vi "Main Page.vi"(8 "error in (no error)":errorcluster, 11 "Node Ptr":T3 format="%.0x") -> (0 "error out":errorcluster)   [LabVIEW 2020, in "FlexRay Custom Device System Explorer.lvlib"]
uses:
  FlexRay Custom Device System Explorer.lvlib
  <vilib>/NI VeriStand/Custom Device API/Custom Device Item Ref.ctl
  Shared/FRConfig.ctl
  Shared/FRInterface.ctl
  Shared/Constants.vi
  <vilib>/NI VeriStand/Custom Device API/Get Item Property (Variant).vi
  <vilib>/NI VeriStand/Custom Device API/Set Item Property (Variant).vi
  <vilib>/NI VeriStand/Custom Device API/Custom Device API.lvlib
  Shared/FlexRay Custom Device Shared.lvlib
  <resource>/objmgr/xnet.rc
panel:
  out "Custom Device Version":string
  out "Baud Rate":u64
  in  "FRConfig":T1 {"FlexRay Interface" items=["FlexRay1", "FlexRay2", "FlexRay3", "FlexRay4", "FlexRay5", "FlexRay6", "FlexRay7", "FlexRay8"]}
  in  "Header":cluster{"Section Name":string}={"Section Name"="FlexRay Interface Settings"}
  in  "Description":string
  in  "Name":string
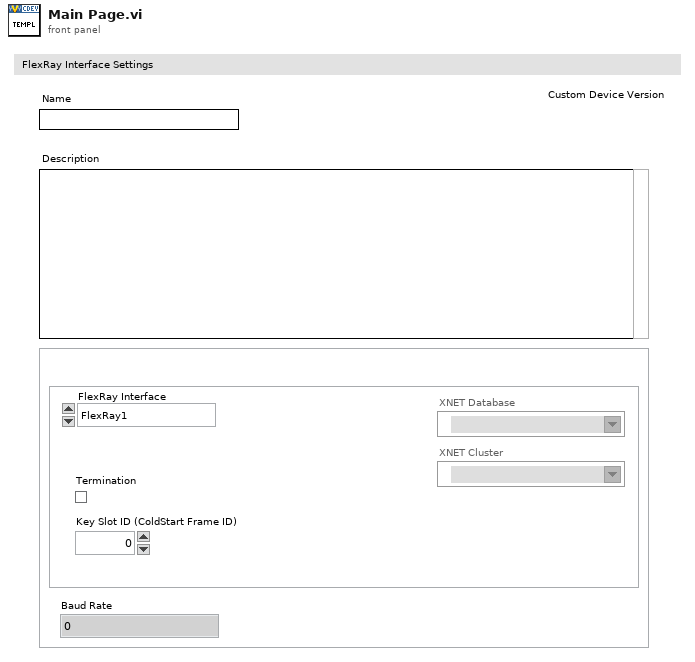
[diagram p1: front panel]
types:
  T1 = typedef "FlexRay Custom Device Shared.lvlib/FRConfig.ctl" = cluster{"FlexRay Interface":T2, "XNET Database":refnum<k21>, "XNET Cluster":refnum<k21>, "ColdStart ID":u32, "Termination":bool}
  T2 = typedef "FlexRay Custom Device Shared.lvlib/FRInterface.ctl" = u16
  T3 = typedef "Custom Device API.lvlib/Custom Device Item Ref.ctl" = u64
  T4 = typedef "Custom Device API.lvlib/Custom Device Item Info.ctl" = cluster{"Name":string, "Is Channel":bool, "GUID":string, "Is Waveform":bool}
  T5 = typedef "Custom Device API.lvlib/Custom Device Commands.ctl" = enum16{"Default", "Item renamed", "Shutdown", "Dynamic button pressed"}
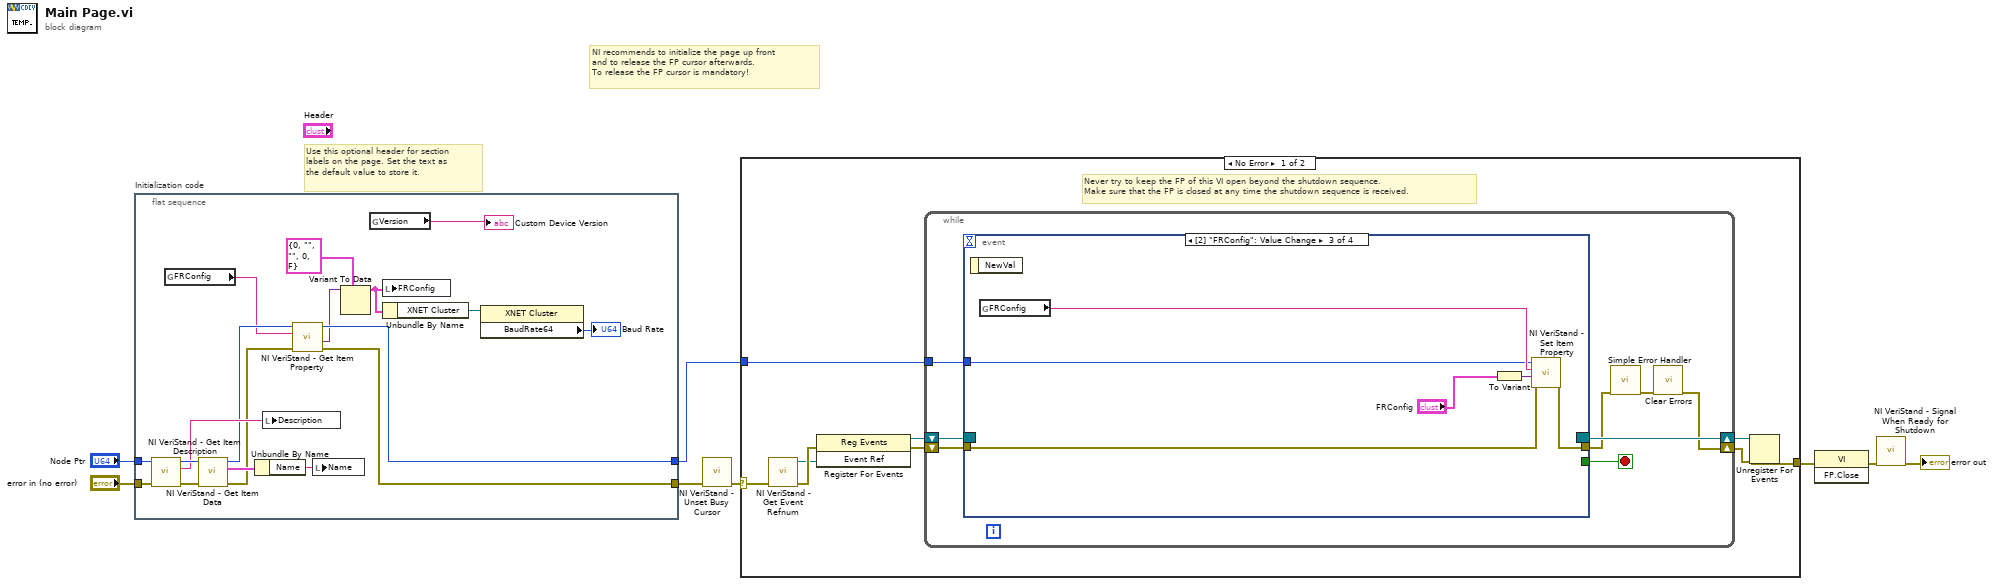
[diagram p0: block diagram]
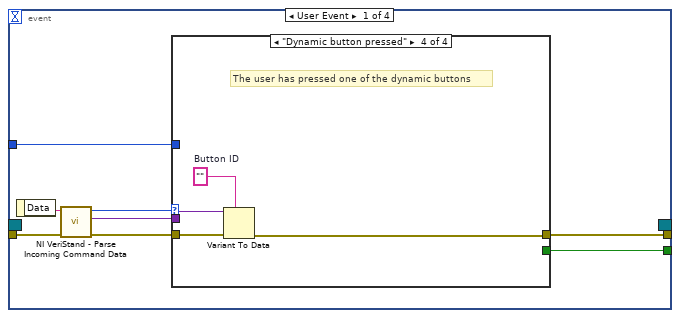
[diagram p2: hidden frame]
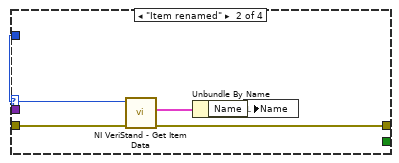
[diagram p4: hidden frame]
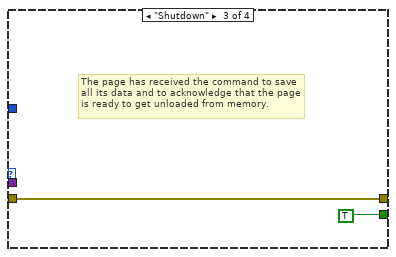
[diagram p5: hidden frame]
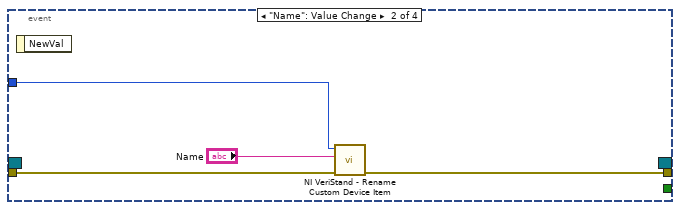
[diagram p6: hidden frame]
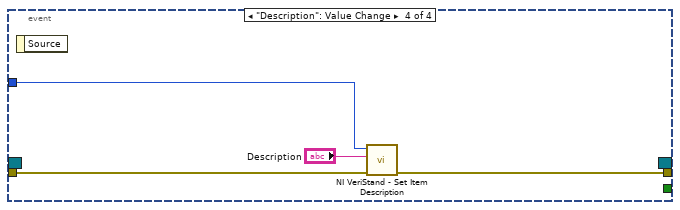
[diagram p7: hidden frame]
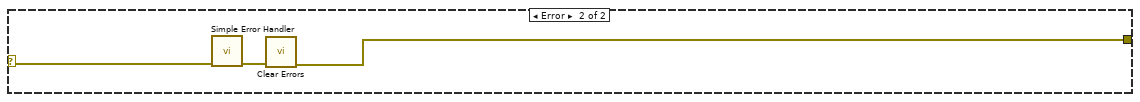
[diagram p8: hidden frame]
diagram:
  # "Use this optional header for section labels on the page. Set the text as the default value to store it."
  # "NI recommends to initialize the page up front\nand to release the FP cursor afterwards.\nTo release the FP cursor is mandatory!"
  n1 = flat-sequence "Initialization code" {
    tunnel: "error in (no error)" -> [w25]
    tunnel: "Node Ptr" -> [w24]
    tunnel: [w16] -> w4
    tunnel: [w18] -> w1
    frame #0 {
      n2 = call <vilib>:"NI VeriStand - Get Item Description.vi"("error in (no error)"=w25, "Item Ref in"=w24) -> ("error out"=w22:errorcluster, "Description"=w23:string, "Item Ref out"=w26:T3)  [unwired: 7 out]
      n3 = global read "Constants.vi" "FRConfig"() -> (w15:string)
      n4 = call <vilib>:"NI VeriStand - Get Item Data.vi"("error in (no error)"=w22, "Item Ref in"=w26) -> ("error out"=w17:errorcluster, "Item Info"=w21:T4, "Item Ref out"=w19:T3)  [unwired: 7 out]
      n5 = Unbundle By Name(w21) -> ("Name"=w20:string)
      n6 = local write "Description"(w23) -> ()
      n7 = call-poly <vilib>:"NI VeriStand - Get Item Property.vi"("error in (no error)"=w17, "Property Name"=w15, "Item Ref in"=w19) -> ("error out"=w16:errorcluster, "Value"=w14:variant, "Item Ref out"=w18:T3)  [unwired: 5 in, 1 out]
      n8 = local write "Name"(w20) -> ()
      n9 = Variant To Data(type=T1 {"FlexRay Interface"=0, "XNET Database"="", "XNET Cluster"="", "ColdStart ID"=0, "Termination"=FALSE} ("FRConfig"), Variant=w14) -> (data=w12:T1)  [unwired: 1 in, 1 out]
      n10 = global read "Constants.vi" "Version"() -> (→"Custom Device Version":string)
      n11 = local write "FRConfig"(w12) -> ()
      n12 = Unbundle By Name(w12) -> ("XNET Cluster"=w11:refnum<k21>)
      n13 = property class="XNET Cluster"(reference=w11) -> ("BaudRate64"=→"Baud Rate":u64)  [unwired: 1 in, 2 out]
    }
  }
  n14 = call <vilib>:"NI VeriStand - Unset Busy Cursor.vi"("error in (no error)"=w4) -> ("error out"=w3:errorcluster)  [unwired: 10 out]
  n15 = case shown="No Error" w3 {
    selector: w3 -> [w27 w80]
    tunnel: [w32 w78] -> w8
    tunnel: w1 -> [w28 _]
    frame No Error {
      # "Never try to keep the FP of this VI open beyond the shutdown sequence.\nMake sure that the FP is closed at any time the shutdown sequence is received."
      n16 = call <vilib>:"NI VeriStand - Get Event Refnum.vi"("error in (no error)"=w27) -> ("error out"=w35:errorcluster, "Event Ref"=w31:refnum<user-event>)  [unwired: 9 out]
      n17 = register-events(error in=w35, w31) -> (reference out=w29:refnum<event-registration>, error out=w30:errorcluster)  [unwired: 1 in]
      n18 = while {
        tunnel: w28 -> [w39]
        shift-right: [w36] -> w33
        shift-left: w30 -> [w42]
        shift-right: [w43] -> w34
        shift-left: w29 -> [w41]
        stop <- w40 stop-if-true
        n19 = event shown="[2] \"FRConfig\": Value Change" {
          selector: w41 -> [_ _ _ _]
          dyn-events: [_ _ _ _] -> w43
          timeout: _ -> [_ _ _ _]
          tunnel: w42 -> [w51 w67 w68 w76]
          tunnel: [w47 _ _ _] -> w40
          tunnel: [w46 w66 w69 w75] -> w38
          tunnel: w39 -> [w45 w65 w70 w77]
          event User Event {
            n20 = event-data() -> ("Data"=w50:string)  [unwired: 1 out]
            n21 = call <vilib>:"NI VeriStand - Parse Incoming Command Data.vi"("error in (no error)"=w51, "Incoming data"=w50) -> ("error out"=w49:errorcluster, "Outgoing data"=w44:variant, "Action"=w48:T5)  [unwired: 7 out]
            n22 = case shown="\"Dynamic button pressed\"" w48 {
              tunnel: w49 -> [w52 w57 w58 w63]
              tunnel: [_ _ TRUE _] -> w47
              tunnel: [w52 w54 w58 w60] -> w46
              tunnel: w45 -> [_ w56 _ _]
              tunnel: w44 -> [_ _ _ w62]
              frame "Default", Default {
              }
              frame "Item renamed" {
                n23 = call <vilib>:"NI VeriStand - Get Item Data.vi"("error in (no error)"=w57, "Item Ref in"=w56) -> ("error out"=w54:errorcluster, "Item Info"=w55:T4)  [unwired: 8 out]
                n24 = Unbundle By Name(w55) -> ("Name"=w53:string)
                n25 = local write "Name"(w53) -> ()
              }
              frame "Shutdown" {
                # "The page has received the command to save all its data and to acknowledge that the page is ready to get unloaded from memory."
              }
              frame "Dynamic button pressed" {
                w61 = ""  # Button ID
                # "The user has pressed one of the dynamic buttons"
                n26 = Variant To Data(error in=w63, type=w61, Variant=w62) -> (error out=w60:errorcluster)  [unwired: 1 out]
              }
            }
          }
          event "Name": Value Change {
            n27 = event-data() -> ()  [unwired: 2 out]
            n28 = call <vilib>:"NI VeriStand - Rename Custom Device Item.vi"("error in (no error)"=w67, "New Name"="Name", "Item Ref in"=w65) -> ("error out"=w66:errorcluster)  [unwired: 1 in, 7 out]
          }
          event Value Change {
            n29 = event-data() -> ()  [unwired: 2 out]
            n30 = global read "Constants.vi" "FRConfig"() -> (w73:string)
            n31 = To Variant(anything="FRConfig") -> (Variant=w72:variant)
            n32 = call-poly <vilib>:"NI VeriStand - Set Item Property.vi"("error in (no error)"=w68, "Value"=w72, "Property Name"=w73, "Item Ref in"=w70) -> ("error out"=w69:errorcluster)  [unwired: 5 in, 2 out]
          }
          event "Description": Value Change {
            n33 = event-data() -> ()  [unwired: 2 out]
            n34 = call <vilib>:"NI VeriStand - Set Item Description.vi"("error in (no error)"=w76, "Description"="Description", "Item Ref in"=w77) -> ("error out"=w75:errorcluster)  [unwired: 8 out]
          }
        }
        n35 = call <vilib>:"Simple Error Handler.vi"("error in (no error)"=w38) -> ("error out"=w37:errorcluster)  [unwired: 1 in, 7 out]
        n36 = call <vilib>:"Clear Errors.vi"("error in (no error)"=w37) -> ("error out"=w36:errorcluster)  [unwired: 1 in, 5 out]
      }
      n37 = Unregister For Events(event registration refnum=w34, error in=w33) -> (error out=w32:errorcluster)
    }
    frame Error {
      n38 = call <vilib>:"Simple Error Handler.vi"("error in (no error)"=w80) -> ("error out"=w79:errorcluster)  [unwired: 1 in, 7 out]
      n39 = call <vilib>:"Clear Errors.vi"("error in (no error)"=w79) -> ("error out"=w78:errorcluster)  [unwired: 1 in, 5 out]
    }
  }
  n40 = invoke class="VI" method="FP.Close"(error in=w8) -> (error out=w7:errorcluster)  [unwired: 2 in, 2 out]
  n41 = call <vilib>:"NI VeriStand - Signal When Ready for Shutdown.vi"("error in (no error)"=w7) -> ("error out"=→"error out":errorcluster)  [unwired: 10 out]
